vi "SGUI Example - demo 2 subpanel.vi"(8 "error in (no error)":errorcluster) -> (0 "error out":errorcluster)   [LabVIEW 2013, in "varilib.lvlib"]
doc: "SGUI lib demo subpanel.\nIt demonstrates handling another panel controls."
uses:
  varilib.lvlib
  SGUI Assign References Mode.ctl
  SGUI Set Single Integer By Label.vi
panel:
  out "random":dbl format="%#_9g"
  in  "btn done":bool
  # "To exit:\n - press STOP on main panel or\n - press done on this panel\n\nSGUI lib reponds to both"
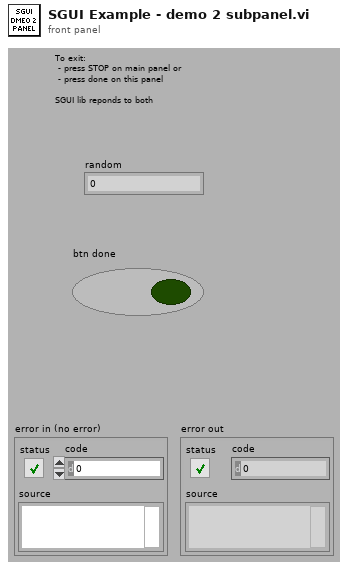
[diagram p1: front panel]
types:
  T1 = typedef "varilib.lvlib/SGUI Assign References Mode.ctl" = enum16{"Add to stack", "Overwrite", "Release last"}
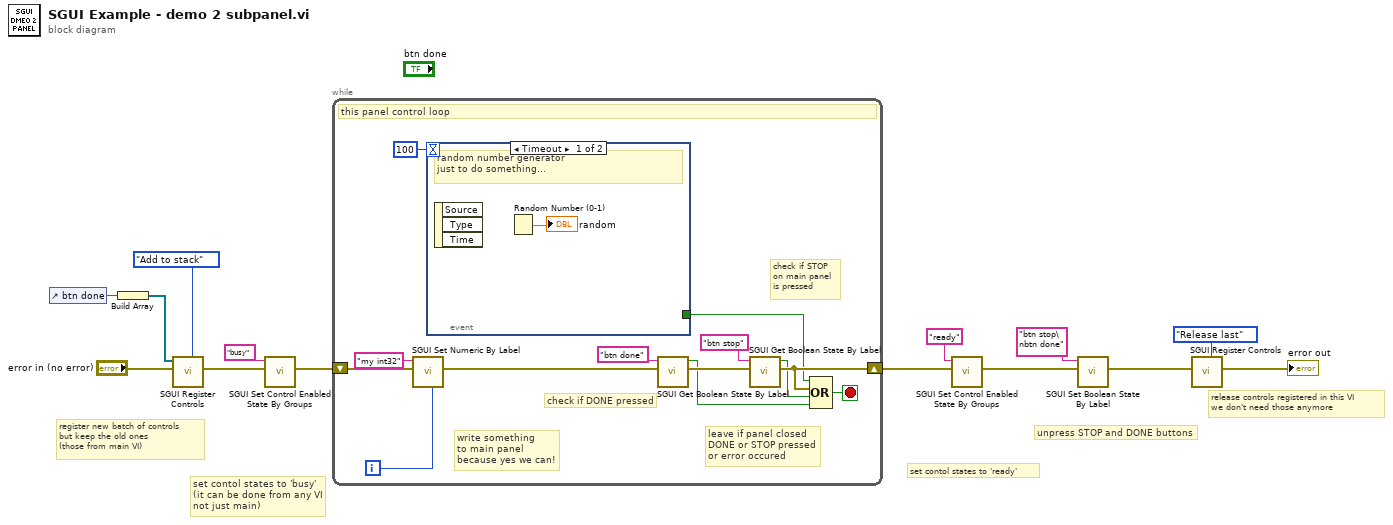
[diagram p0: block diagram]
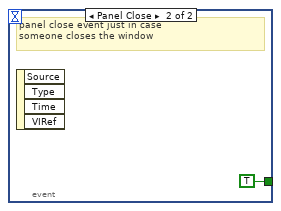
[diagram p2: hidden frame]
diagram:
  # "release controls registered in this VI\nwe don't need those anymore"
  # "set contol states to 'ready'"
  # "set contol states to 'busy'\n(it can be done from any VI\nnot just main)"
  # "unpress STOP and DONE buttons"
  # "register new batch of controls\nbut keep the old ones\n(those from main VI)"
  n1 = control-ref of="btn done"() -> (w12:refnum<vi>)
  n2 = Build Array(w12) -> (w11:refnum<vi>[])
  n3 = call "SGUI Register Controls.vi"("error in"="error in (no error)", "control references (empty)"=w11, "register mode (overwrite)"=SGUI_Assign_References_Mode."Add to stack") -> ("error out"=w9:errorcluster)  [unwired: 7 in, 1 out]
  n4 = call "SGUI Set Control Enabled State By Groups.vi"("error in"=w9, "group name to enable (none)"="busy") -> ("error out"=w8:errorcluster)  [unwired: 8 in, 1 out]
  n5 = while {
    shift-right: [w25] -> w6
    shift-left: w8 -> [w18]
    i -> [w15]
    stop <- w23 stop-if-true
    # "write something\nto main panel\nbecause yes we can!"
    # "leave if panel closed\nDONE or STOP pressed\nor error occured"
    # "check if STOP\non main panel\nis pressed"
    # "check if DONE pressed"
    # "this panel control loop"
    n6 = call-poly "SGUI Set Numeric By Label.vi"("error in"=w18, "label (empty)"="my int32", "value (none)"=w15) -> ("error out"=w17:errorcluster)  [unwired: 7 in, 1 out]
    n7 = event shown="[0] Timeout" {
      selector: _ -> [_ _]
      dyn-events: _ -> [_ _]
      timeout: 100 -> [_ _]
      tunnel: [_ TRUE] -> w22
      event Timeout {
        # "random number generator\njust to do something..."
        n8 = event-data() -> ()  [unwired: 1 in, 3 out]
        n9 = Random Number (0-1)() -> (number: 0 to 1=→"random":dbl)
      }
      event Panel Close {
        # "panel close event just in case\nsomeone closes the window"
        n10 = event-data() -> ()  [unwired: 1 in, 4 out]
      }
    }
    n11 = call "SGUI Get Boolean State By Label.vi"("error in"=w17, "control label ('btn stop')"="btn done") -> ("error out"=w20:errorcluster, "binary state out"=w19:bool)  [unwired: 7 in, 1 out]
    n12 = call "SGUI Get Boolean State By Label.vi"("error in"=w20, "control label ('btn stop')"="btn stop") -> ("error out"=w25:errorcluster, "binary state out"=w24:bool)  [unwired: 7 in, 1 out]
    n13 = Compound Arithmetic op=OR(w22, w25, w24, w19) -> (w23:bool)
  }
  n14 = call "SGUI Set Control Enabled State By Groups.vi"("error in"=w6, "group name to enable (none)"="ready") -> ("error out"=w5:errorcluster)  [unwired: 8 in, 1 out]
  n15 = call "SGUI Set Boolean State By Label.vi"("error in"=w5, "control label(s) ('btn stop')"="btn stop\nbtn done") -> ("error out"=w3:errorcluster)  [unwired: 8 in, 1 out]
  n16 = call "SGUI Register Controls.vi"("error in"=w3, "register mode (overwrite)"=SGUI_Assign_References_Mode."Release last") -> ("error out"=→"error out":errorcluster)  [unwired: 8 in, 1 out]
